vi "2021_day1_task2.vi"() -> ()   [LabVIEW 2021]
panel:
  out "Array":i32[](array[numeric])
  out "Numeric 2":i32
  out "Numeric":i32
  out "array":i32[](array[numeric])
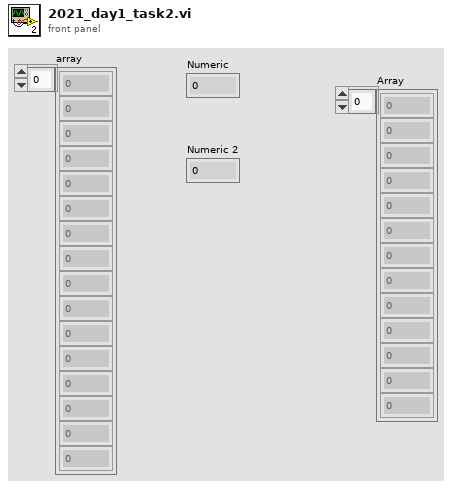
[diagram p1: front panel]
diagram:
  (unwired) "199\n200\n208\n210\n200\n207\n240\n269\n260\n263" ("format string")
  n1 = Spreadsheet String To Array(delimiter (Tab)="\n", format string="%d", spreadsheet string="193\n197\n188\n170\n162\n180\n183\n211\n213\n235\n238\n237\n234\n227\n222\n221\n223\n224\n223\n216\n217\n226\n234\n228\n230\n237\n239\n242\n244\n246\n242\n258\n269\n270\n255\n257\n261\n262\n258\n257\n262\n261\n260\n263\n266\n282\n281\n290\n299\n300\n302\n288\n286\n296\n293\n292\n272\n270\n283\n294\n311\n310\n309\n310\n312\n314\n318\n330\n331\n332\n344\n342\n328\n317\n314\n310\n306\n310\n351\n353\n352\n354\n355\n349\n350\n354\n353\n352\n357\n362\n358\n346\n329\n322\n320\n294\n277\n270\n273\n275\n283\n279\n277\n271\n273\n246\n247\n248\n255\n258\n243\n267\n266\n282\n281\n282\n284\n288\n290\n289\n288\n298\n302\n299\n300\n303\n297\n324\n325\n329\n332\n313\n309\n307\n299\n289\n315\n320\n311\n295\n303\n307\n329\n330\n329\n317\n318\n334\n335\n310\n...", array type (2D Dbl)=i32[] []) -> (array=w6:i32[])
  "array" <- w6
  n2 = Array Size(array=w6) -> (size(s)=w5:i32)
  n3 = Subtract(x=w5, y=2) -> (x-y=w4:i32)
  n4 = for {
    tunnel: w6 -> [w16] mode=indexing
    tunnel: w6 -> [w18]
    shift-right: [w14] -> w9
    shift-left: 0 -> [w15]
    i -> [w17]
    n5 = case shown="Default" w17 {
      tunnel: w18 -> [_ w27]
      tunnel: w17 -> [_ w26]
      tunnel: w16 -> [_ w23]
      tunnel: w15 -> [w19 w20]
      tunnel: [w19 w21] -> w14
      frame 0 {
      }
      frame Default {
        n6 = Decrement(x=w26) -> (x-1=w25:i32)
        n7 = Index Array(array=w27, index=w25) -> (element=w24:i32)
        n8 = Greater?(x=w23, y=w24) -> (0:w22:bool)
        n9 = case shown="True" w22 {
          tunnel: [w28 w29] -> w21
          tunnel: w20 -> [w28 w30]
          frame False {
          }
          frame True {
            n10 = Increment(x=w30) -> (x+1=w29:i32)
          }
        }
      }
    }
  }
  "Numeric" <- w9
  n11 = for {
    N: w4 -> [_]
    tunnel: w6 -> [w35]
    shift-right: [w36] -> w8
    shift-left: 0 -> [w37]
    shift-right: [w31] -> _
    shift-left: _ -> [w38]
    tunnel: [w31] -> w2 mode=indexing
    i -> [w32]
    n12 = Array Subset(array=w35, index=w32, length=3) -> (w33:i32[])
    n13 = Add Array Elements(numeric array=w33) -> (sum=w31:i32)
    n14 = case shown="Default" w32 {
      tunnel: w38 -> [_ w44]
      tunnel: w37 -> [w39 w43]
      tunnel: [w39 w42] -> w36
      tunnel: w31 -> [_ w40]
      frame 0 {
      }
      frame Default {
        n15 = Greater?(x=w40, y=w44) -> (0:w41:bool)
        n16 = case shown="True" w41 {
          tunnel: [w45 w46] -> w42
          tunnel: w43 -> [w45 w47]
          frame False {
          }
          frame True {
            n17 = Increment(x=w47) -> (x+1=w46:i32)
          }
        }
      }
    }
  }
  "Numeric 2" <- w8
  "Array" <- w2
